vi "Proceed.vi"(7 "component is ready (Y)":bool=TRUE, 8 "error in (no error)":errorcluster, 10 "ProceedMessage":refnum<class "ProceedMessage.lvclass">, 11 "Template in":refnum<class "Template.lvclass">) -> (0 "error out":errorcluster, 2 "all observers are ready?":bool, 3 "Template out":refnum<class "Template.lvclass">)   [LabVIEW 2012, in "Template.lvclass"]
doc: "The Proceed method is used to check if your component is ready. Also it checks if the observers are ready. When the observers and the component are ready, it sends the proceed to its observee. If it's the highest observee, it distributes a stop command."
uses:
  Template.lvclass
  <vilib>/Distrio/Murmex/ProceedMessage/ProceedMessage.lvclass
  <vilib>/Distrio/Murmex/Murmex/Murmex.lvclass
panel:
  # "This method is called when the PROCEED\ntrigger is sent. \n\nOverride this method when your component needs to\nrespond to this trigger. \n\nCall parent for proper implementation"
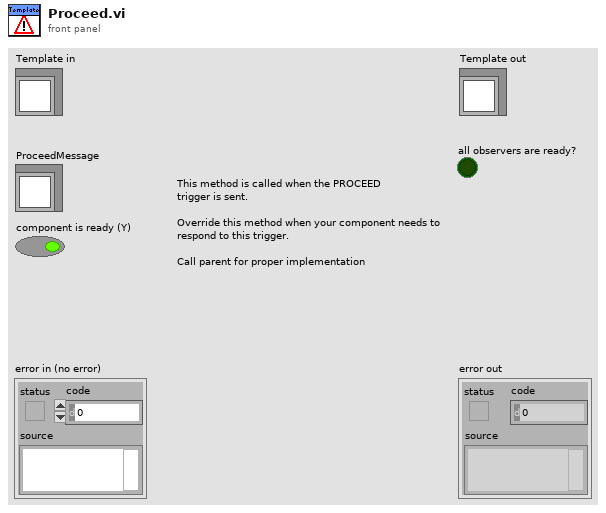
[diagram p1: front panel]
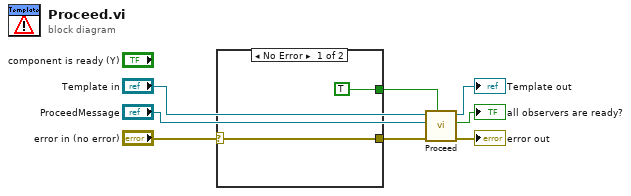
[diagram p0: block diagram]
diagram:
  n1 = case shown="No Error" "error in (no error)" {
    selector: "error in (no error)" -> [w10 w11]
    tunnel: [w10 w11] -> w2
    tunnel: [TRUE _] -> w1
    frame No Error {
    }
    frame Error {
    }
  }
  n2 = call-parent "Proceed.vi"("component is ready (Y)"=w1, "error in (no error)"=w2, "ProceedMessage"="ProceedMessage", "Murmex in"="Template in") -> ("error out"=→"error out":errorcluster, "all observers are ready?"=→"all observers are ready?":bool, "Murmex out"=→"Template out":refnum<class "Template.lvclass">)  [unwired: 5 in]
